vi "Position Zero Key.vi"(8 "error in (no error)":errorcluster, 11 "Zero Key":refnum<vi>) -> (0 "error out":errorcluster)   [LabVIEW 2014]
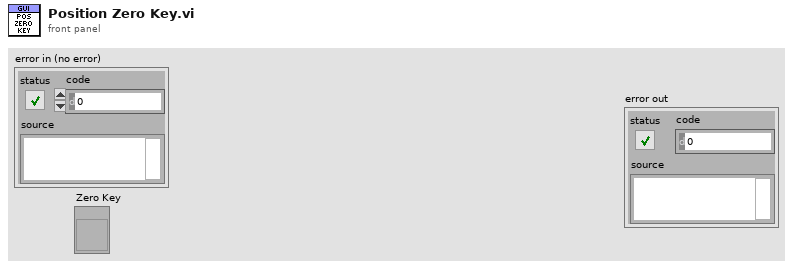
[diagram p1: front panel]
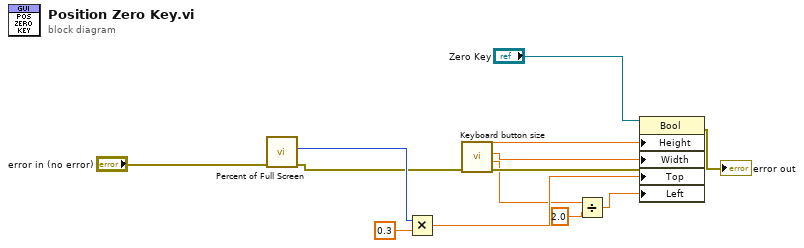
[diagram p0: block diagram]
diagram:
  n1 = call "Percent of Full Screen.vi"("error in (no error)"="error in (no error)") -> ("error out"=w4:errorcluster, "Bottom"=w7:i16)  [unwired: 8 in, 1 out]
  n2 = Multiply(x=w7, y=0.3) -> (x*y=w5:dbl)
  n3 = call "Keyboard button size.vi"("error in (no error)"=w4) -> ("error out"=w12:errorcluster, "Key Spacing"=w3:dbl, "Key Width"=w10:dbl, "Key Height"=w9:dbl)  [unwired: 7 in]
  n4 = Divide(x=w3, y=2.0) -> (x/y=w1:dbl)
  n5 = property class="Bool"(reference="Zero Key", error in=w12, "Height"=w9, "Width"=w10, "Top"=w5, "Left"=w1) -> (error out=→"error out":errorcluster)  [unwired: 1 out]
